vi "Facade.vi"(0 "Data In":T4, 2 "Display State In":T2, 3 "Container State":T3) -> (6 "Data Out":T4, 7 "Display State Out":T2, 8 "Action":T1)   [LabVIEW 2015, in "KNumeric (DBL).xctl"]
uses:
  KNumeric (DBL).xctl
  Data.ctl
  <vilib>/_xctls/Container State.ctl
  State.ctl
  <vilib>/_xctls/Action.ctl
  <vilib>/_xctls/XControlSupport.lvlib
panel:
  in  "Expr":string
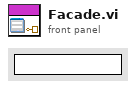
[diagram p1: front panel]
types:
  T1 = typedef "XControlSupport.lvlib/Action.ctl" = cluster{"Data Changed?":bool, "State Changed?":bool, "Action Name":string}
  T2 = typedef "KNumeric (DBL).xctl/State.ctl" = cluster{"mixed":bool, "format":string, "Value":dbl}
  T3 = typedef "XControlSupport.lvlib/Container State.ctl" = cluster{"Indicator?":bool, "Run Mode?":bool, " Refnum":refnum<vi>}
  T4 = typedef "KNumeric (DBL).xctl/Data.ctl" = dbl
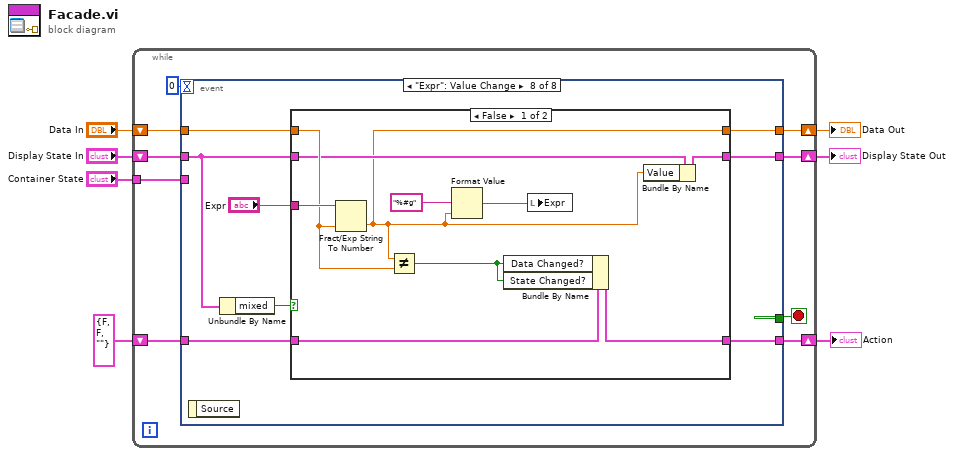
[diagram p0: block diagram]
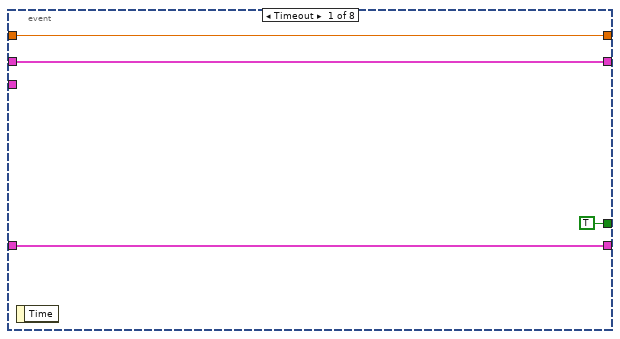
[diagram p2: hidden frame]
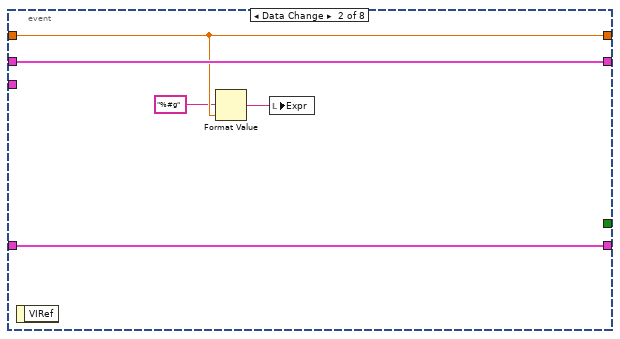
[diagram p3: hidden frame]
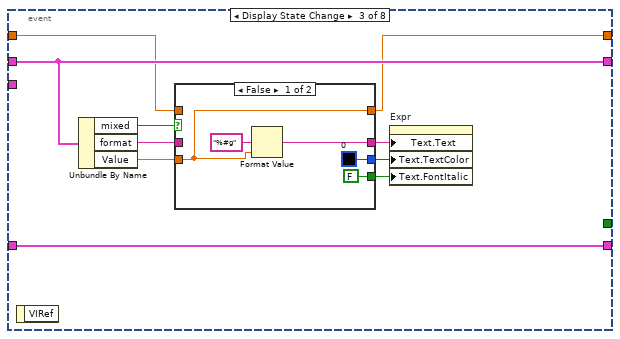
[diagram p4: hidden frame]
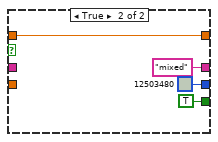
[diagram p5: hidden frame]
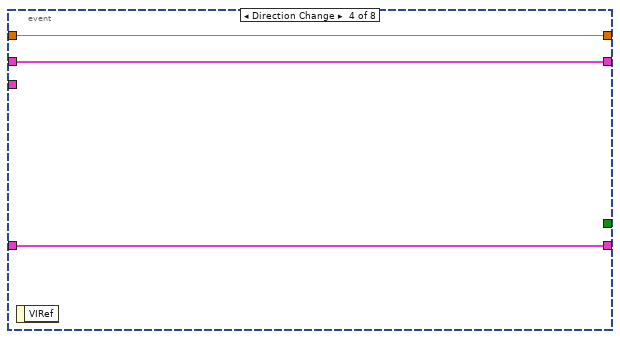
[diagram p6: hidden frame]
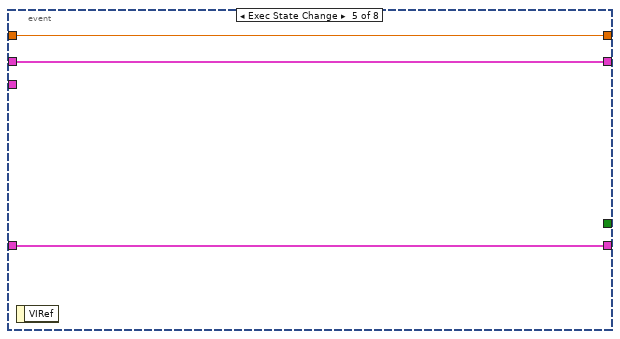
[diagram p7: hidden frame]
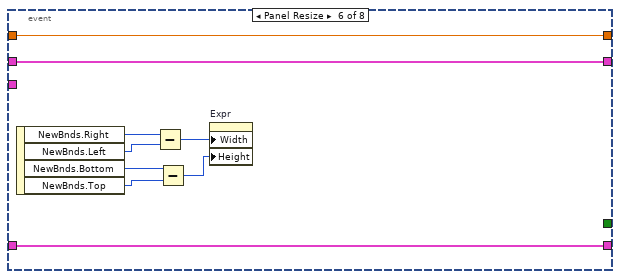
[diagram p8: hidden frame]
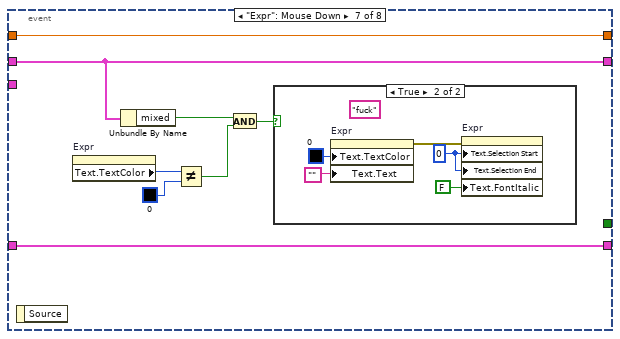
[diagram p9: hidden frame]
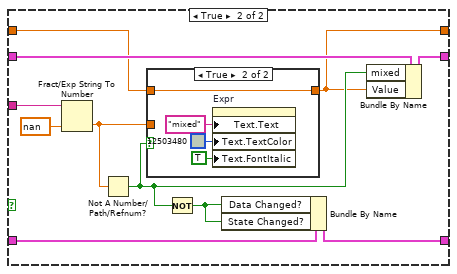
[diagram p11: hidden frame]
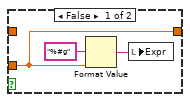
[diagram p12: hidden frame]
diagram:
  n1 = while {
    shift-right: [w15] -> w4
    shift-left: "Display State In" -> [w16]
    tunnel: "Container State" -> [w12]
    shift-right: [w10] -> w7
    shift-left: "Data In" -> [w11]
    shift-right: [w8] -> w2
    shift-left: T1 {"Data Changed?"=FALSE, "State Changed?"=FALSE, "Action Name"=""} ("Action") -> [w9]
    stop <- w14 stop-if-true
    n2 = event shown="[7] \"Expr\": Value Change" {
      selector: _ -> [_ _ _ _ _ _ _ _]
      dyn-events: _ -> [_ _ _ _ _ _ _ _]
      timeout: 0 -> [_ _ _ _ _ _ _ _]
      tunnel: w16 -> [w18 w24 w34 w47 w50 w59 w66 w75]
      tunnel: [w18 w24 w34 w47 w50 w59 w66 w73] -> w15
      tunnel: [TRUE _ _ _ _ _ _ _] -> w14
      tunnel: w12 -> [_ _ _ _ _ _ _ _]
      tunnel: w11 -> [w17 w23 w31 w46 w49 w58 w64 w77]
      tunnel: [w17 w23 w26 w46 w49 w58 w64 w76] -> w10
      tunnel: [w19 w25 w35 w45 w48 w57 w67 w79] -> w8
      tunnel: w9 -> [w19 w25 w35 w45 w48 w57 w67 w80]
      event Timeout {
        n3 = event-data() -> ()  [unwired: 1 in, 1 out]
      }
      event Data Change {
        n4 = event-data() -> ()  [unwired: 1 in, 1 out]
        n5 = Format Value(format string="%#g", value (0)=w23) -> (output string=w22:string)  [unwired: 1 in]
        n6 = local write "Expr"(w22) -> ()
      }
      event Display State Change {
        n7 = event-data() -> ()  [unwired: 1 in, 1 out]
        n8 = Unbundle By Name(w34) -> ("mixed"=w33:bool, "format"=w32:string, "Value"=w27:dbl)
        n9 = case shown="False" w33 {
          tunnel: w32 -> [_ _]
          tunnel: w31 -> [_ w41]
          tunnel: [w40 "mixed" ("output string")] -> w30
          tunnel: [u32 0 u32 12503480] -> w29
          tunnel: [FALSE TRUE] -> w28
          tunnel: w27 -> [w36 _]
          tunnel: [w36 w41] -> w26
          frame False {
            n10 = Format Value(format string="%#g", value (0)=w36) -> (output string=w40:string)  [unwired: 1 in]
          }
          frame True {
          }
        }
        n11 = property on="Expr" class="Str"("Text.Text"=w30, "Text.TextColor"=w29, "Text.FontItalic"=w28) -> ()  [unwired: 2 in, 2 out]
      }
      event Direction Change {
        n12 = event-data() -> ()  [unwired: 1 in, 1 out]
      }
      event Exec State Change {
        n13 = event-data() -> ()  [unwired: 1 in, 1 out]
      }
      event Panel Resize {
        n14 = event-data() -> ("NewBnds.Right"=w56:i16, "NewBnds.Left"=w54:i16, "NewBnds.Bottom"=w53:i16, "NewBnds.Top"=w52:i16)  [unwired: 1 in]
        n15 = Subtract(x=w56, y=w54) -> (x-y=w55:i16)
        n16 = Subtract(x=w53, y=w52) -> (x-y=w51:i16)
        n17 = property on="Expr" class="Str"("Width"=w55, "Height"=w51) -> ()  [unwired: 2 in, 2 out]
      }
      event "Expr": Mouse Down {
        n18 = event-data() -> ()  [unwired: 1 in, 1 out]
        n19 = property on="Expr" class="Str"() -> ("Text.TextColor"=w63:u32)  [unwired: 2 in, 2 out]
        n20 = Unbundle By Name(w66) -> ("mixed"=w65:bool)
        n21 = Not Equal?(x=w63, y=u32 0) -> (x != y?=w60:bool)
        n22 = And(x=w65, y=w60) -> (x .and. y?=w61:bool)
        n23 = case shown="True" w61 {
          frame False {
          }
          frame True {
            w68 = u32 0 ("Text.Selection:Start")
            (unwired) "fuck"
            n24 = property on="Expr" class="Str"("Text.TextColor"=u32 0, "Text.Text"="") -> (error out=w71:errorcluster)  [unwired: 2 in, 1 out]
            n25 = property on="Expr" class="Str"(error in=w71, "Text.Selection Start"=w68, "Text.Selection End"=w68, "Text.FontItalic"=FALSE ("Text.Font:Italic")) -> ()  [unwired: 1 in, 2 out]
          }
        }
      }
      event "Expr": Value Change {
        n26 = event-data() -> ()  [unwired: 1 in, 1 out]
        n27 = Unbundle By Name(w75) -> ("mixed"=w74:bool)
        n28 = case shown="False" w74 {
          tunnel: w80 -> [w90 w101]
          tunnel: [w89 w100] -> w79
          tunnel: "Expr" -> [w86 w99]
          tunnel: w77 -> [w85 w93]
          tunnel: [w82 w91] -> w76
          tunnel: w75 -> [w84 w98]
          tunnel: [w83 w97] -> w73
          frame False {
            n29 = Fract/Exp String To Number(string=w86, default (0 dbl)=w85) -> (number=w82:dbl)  [unwired: 2 in, 1 out]
            n30 = Not Equal?(x=w82, y=w85) -> (x != y?=w81:bool)
            n31 = Format Value(format string="%#g", value (0)=w82) -> (output string=w87:string)  [unwired: 1 in]
            n32 = Bundle By Name(cluster=w90, "Data Changed?"=w81, "State Changed?"=w81) -> (w89:T1)
            n33 = local write "Expr"(w87) -> ()
            n34 = Bundle By Name(cluster=w84, "Value"=w82) -> (w83:T2)
          }
          frame True {
            n35 = Fract/Exp String To Number(string=w99, default (0 dbl)=nan) -> (number=w95:dbl)  [unwired: 2 in, 1 out]
            n36 = Not A Number/Path/Refnum?(number/path/refnum=w95) -> (NaN/Path/Refnum?=w92:bool)
            n37 = case shown="True" w92 {
              tunnel: w95 -> [w102 _]
              tunnel: w93 -> [_ w108]
              tunnel: [w102 w108] -> w91
              frame False {
                n38 = Format Value(format string="%#g", value (0)=w102) -> (output string=w103:string)  [unwired: 1 in]
                n39 = local write "Expr"(w103) -> ()
              }
              frame True {
                n40 = property on="Expr" class="Str"("Text.Text"="mixed" ("output string"), "Text.TextColor"=u32 12503480, "Text.FontItalic"=TRUE) -> ()  [unwired: 2 in, 2 out]
              }
            }
            n41 = Not(x=w92) -> (.not. x?=w94:bool)
            n42 = Bundle By Name(cluster=w101, "Data Changed?"=w94, "State Changed?"=w94) -> (w100:T1)
            n43 = Bundle By Name(cluster=w98, "mixed"=w92, "Value"=w91) -> (w97:T2)
          }
        }
      }
    }
  }
  "Display State Out" <- w4
  "Data Out" <- w7
  "Action" <- w2
